vi "Log.vi"(7 "Log Level":T1, 8 "error in (no error)":errorcluster, 9 "Message":string, 10 "Source":string, 11 "AppLogger in":refnum<class "AppLogger.lvclass">) -> (0 "error out":errorcluster, 3 "AppLogger out":refnum<class "AppLogger.lvclass">)   [LabVIEW 2014, in "AppLogger.lvclass"]
uses:
  AppLogger.lvclass
  Message.Log/Enum.LogLevel.ctl
  AppLogger.Message.Log.lvclass
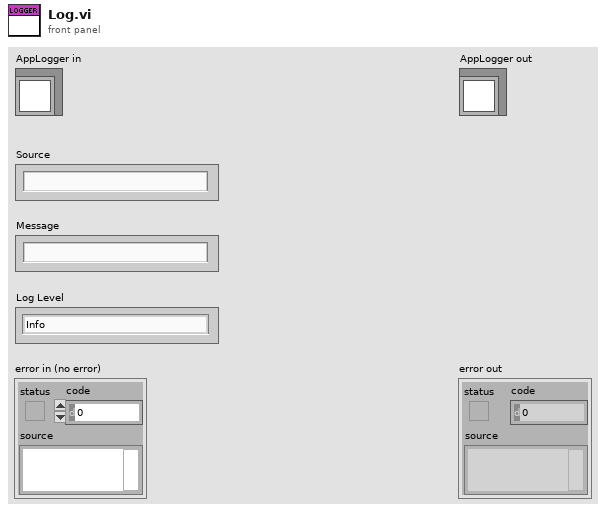
[diagram p1: front panel]
types:
  T1 = typedef "AppLogger.Message.Log.lvclass/Enum.LogLevel.ctl" = enum16{"Info", "Warning", "Small Error", "Fatal Error"}
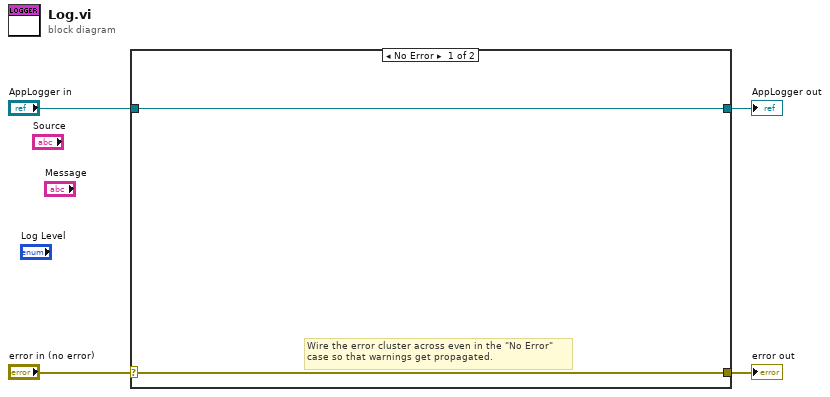
[diagram p0: block diagram]
diagram:
  n1 = case shown="No Error" "error in (no error)" {
    selector: "error in (no error)" -> [w5 w8]
    tunnel: [w5 w8] -> w3
    tunnel: [w6 w7] -> w1
    tunnel: "AppLogger in" -> [w6 w7]
    frame No Error {
      # "Wire the error cluster across even in the \"No Error\"\ncase so that warnings get propagated."
    }
    frame Error {
    }
  }
  "error out" <- w3
  "AppLogger out" <- w1
